vi "ConsolidatedLimitSwitchMotors.vi"(4 "Start at bottom?":bool=TRUE, 6 "BackwardValue":dbl=-0.10000000000000014 min=-1.0 max=0.0 step=0.1, 7 "ForwardValue":dbl=0.10000000000000014 min=0.0 max=1.0 step=0.1, 8 "CurrentLSValue":bool, 9 "UsingEncoder?":bool, 10 "AngleEncoderValue":dbl, 11 "CurrentInput":dbl) -> (0 "New Output":dbl)   [LabVIEW 2013]
uses:
  LimitSwitchState.ctl
panel:
  in  "ScaleFactor":dbl=2.0
  in  "SlowDownTol":dbl=1.0
  in  "HalfWayAngle":dbl=30.0
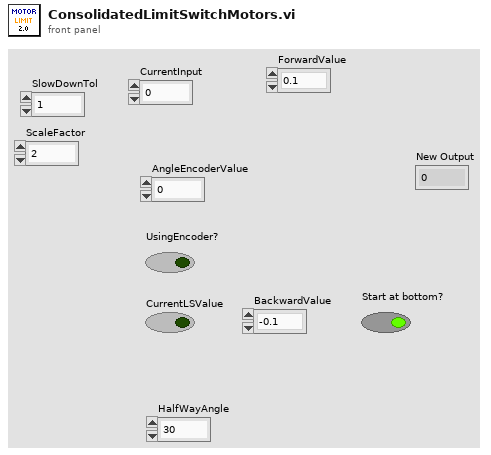
[diagram p1: front panel]
types:
  T1 = typedef "LimitSwitchState.ctl" = enum16{"Normal", "TopLS", "BottomLS", "Begin"}
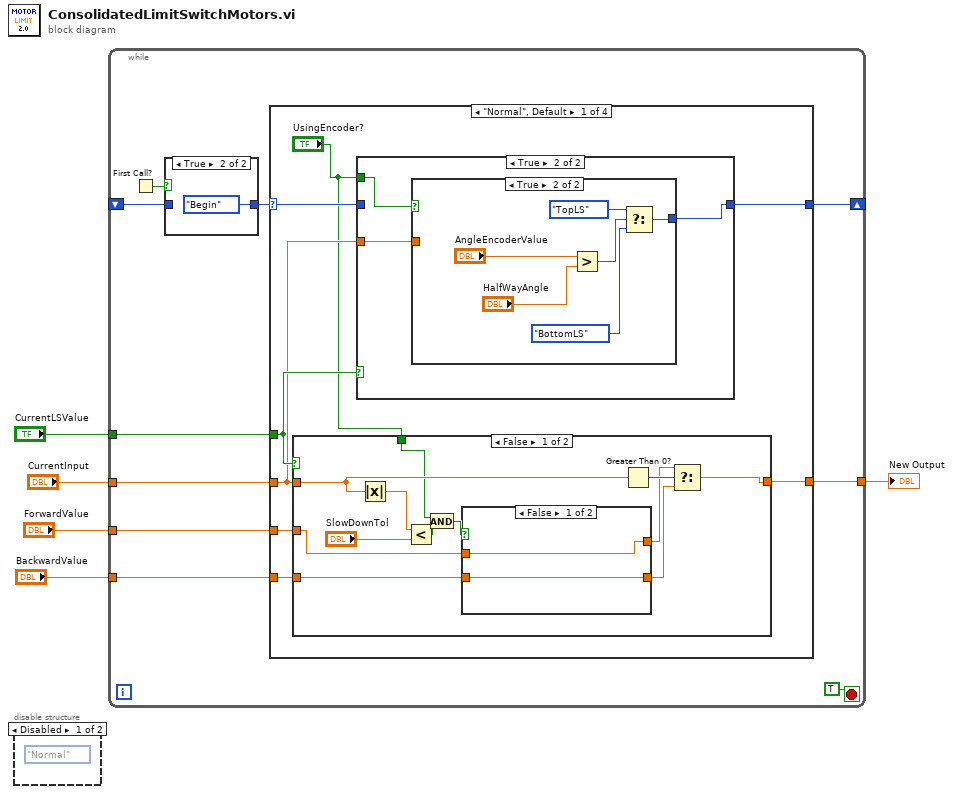
[diagram p0: block diagram]
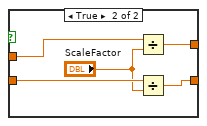
[diagram p4: hidden frame]
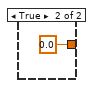
[diagram p5: hidden frame]
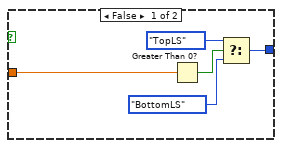
[diagram p7: hidden frame]
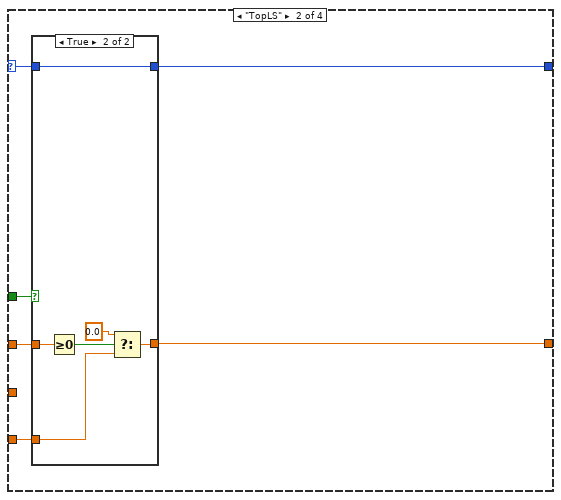
[diagram p8: hidden frame]
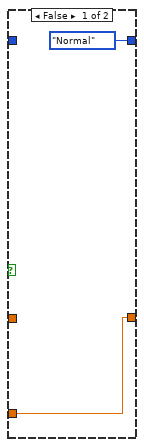
[diagram p9: hidden frame]
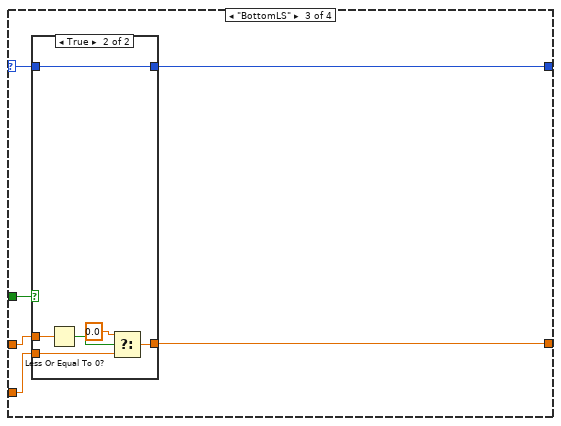
[diagram p10: hidden frame]
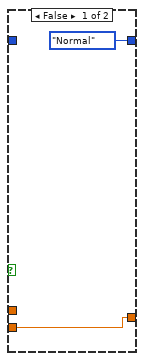
[diagram p11: hidden frame]
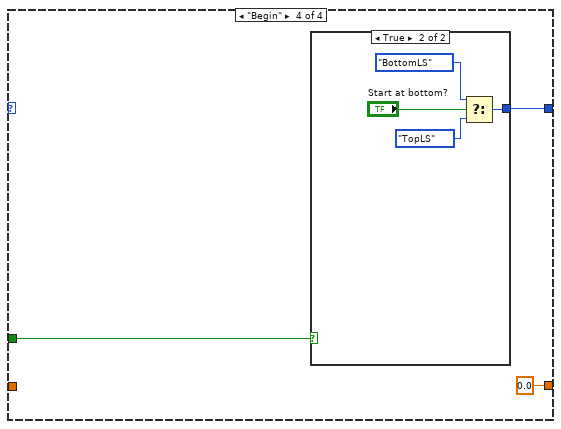
[diagram p12: hidden frame]
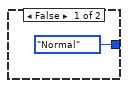
[diagram p13: hidden frame]
diagram:
  n1 = disable-structure shown="Disabled" {
    frame Disabled {
      (unwired) LimitSwitchState."Normal" ("f")
    }
    frame Enabled {
    }
  }
  n2 = while {
    tunnel: "CurrentInput" -> [w15]
    tunnel: "CurrentLSValue" -> [w14]
    tunnel: [w13] -> w3
    tunnel: "BackwardValue" -> [w12]
    tunnel: "ForwardValue" -> [w11]
    shift-right: [w9] -> _
    shift-left: _ -> [w7]
    stop <- TRUE stop-if-true
    n3 = First Call?() -> (First Call?: T/F=w8:bool)
    n4 = case shown="True" w8 {
      tunnel: [w16 LimitSwitchState."Begin" ("f")] -> w6
      tunnel: w7 -> [w16 _]
      frame False {
      }
      frame True {
      }
    }
    n5 = case shown="\"Normal\", Default" w6 {
      selector: w6 -> [w25 w65 w79 _]
      tunnel: w15 -> [w19 w64 w76 _]
      tunnel: w14 -> [w20 w66 w80 w89]
      tunnel: [w21 w63 w77 0.0 ("ForwardValue")] -> w13
      tunnel: w12 -> [w22 w61 _ _]
      tunnel: w11 -> [w23 _ w75 _]
      tunnel: [w24 w62 w78 w91] -> w9
      frame "Normal", Default {
        n6 = case shown="False" w20 {
          tunnel: w23 -> [w35 _]
          tunnel: w22 -> [w34 _]
          tunnel: [w36 0.0 ("BackwardValue")] -> w21
          tunnel: w19 -> [w31 _]
          tunnel: "UsingEncoder?" -> [w26 _]
          frame False {
            n7 = Absolute Value(x=w31) -> (abs(x)=w30:dbl)
            n8 = Less?(x=w30, y="SlowDownTol") -> (x < y?=w28:bool)
            n9 = And(x=w26, y=w28) -> (x .and. y?=w27:bool)
            n10 = case shown="False" w27 {
              tunnel: w35 -> [w39 w44]
              tunnel: w34 -> [w38 w43]
              tunnel: [w38 w42] -> w32
              tunnel: [w39 w41] -> w33
              frame False {
              }
              frame True {
                n11 = Divide(x=w44, y="ScaleFactor") -> (x/y=w41:dbl)
                n12 = Divide(x=w43, y="ScaleFactor") -> (x/y=w42:dbl)
              }
            }
            n13 = Greater Than 0?(x=w31) -> (x > 0?=w37:bool)
            n14 = Select(t=w33, s=w37, f=w32) -> (s? t:f=w36:dbl)
          }
          frame True {
          }
        }
        n15 = case shown="True" w20 {
          tunnel: w25 -> [w46 _]
          tunnel: [w46 w48] -> w24
          tunnel: w19 -> [_ w49]
          tunnel: "UsingEncoder?" -> [_ w47]
          frame False {
          }
          frame True {
            n16 = case shown="True" w47 {
              tunnel: w49 -> [w53 _]
              tunnel: [w52 w55] -> w48
              frame False {
                n17 = Greater Than 0?(x=w53) -> (x > 0?=w54:bool)
                n18 = Select(t=LimitSwitchState."TopLS" ("f"), s=w54, f=LimitSwitchState."BottomLS") -> (s? t:f=w52:T1)
              }
              frame True {
                n19 = Greater?(x="AngleEncoderValue", y="HalfWayAngle") -> (0:w56:bool)
                n20 = Select(t=LimitSwitchState."TopLS" ("f"), s=w56, f=LimitSwitchState."BottomLS") -> (s? t:f=w55:T1)
              }
            }
          }
        }
      }
      frame "TopLS" {
        n21 = case shown="True" w66 {
          tunnel: w65 -> [_ w69]
          tunnel: [LimitSwitchState."Normal" ("f") w69] -> w62
          tunnel: w64 -> [_ w72]
          tunnel: [w67 w71] -> w63
          tunnel: w61 -> [w67 w70]
          frame False {
          }
          frame True {
            n22 = Greater Or Equal To 0?(x=w72) -> (x >= 0?=w74:bool)
            n23 = Select(t=0.0, s=w74, f=w70) -> (s? t:f=w71:dbl)
          }
        }
      }
      frame "BottomLS" {
        n24 = case shown="True" w80 {
          tunnel: w79 -> [_ w83]
          tunnel: [LimitSwitchState."Normal" ("f") w83] -> w78
          tunnel: [w81 w85] -> w77
          tunnel: w76 -> [_ w86]
          tunnel: w75 -> [w81 w84]
          frame False {
          }
          frame True {
            n25 = Less Or Equal To 0?(x=w86) -> (x <= 0?=w88:bool)
            n26 = Select(t=0.0, s=w88, f=w84) -> (s? t:f=w85:dbl)
          }
        }
      }
      frame "Begin" {
        n27 = case shown="True" w89 {
          tunnel: [LimitSwitchState."Normal" ("f") w94] -> w91
          frame False {
          }
          frame True {
            n28 = Select(t=LimitSwitchState."BottomLS" ("f"), s="Start at bottom?", f=LimitSwitchState."TopLS") -> (s? t:f=w94:T1)
          }
        }
      }
    }
  }
  "New Output" <- w3
